vi "Read2 Channels Metodo.vi"(6 "Measurement Type (0: Phase)":i32(ring) items=["Phase", "Delay", "DelayRR", "DelayRF", "DelayFR", "DelayFF"], 8 "error in (no error)":errorcluster, 9 "Channels":T2={"Data Tektronix"={"Channel 1 (1: Channel 1)"=1, "Channel 2 (2: Channel 2)"=2}, "Data Keysight"={"Channels 2"=[], "Timeout (10000 ms)"=10000}} {"Data Keysight"."Channels 2" items=["Channel 1"=0, "Channel 2"=1, "Channel 3"=2, "Channel 4"=3, "Waveform Memory 1"=5, "Waveform Memory 2"=6, "Serial Bus 1"=7, "Serial Bus 2"=8, "Digital Bus Low"=9, "Digital Bus High "=10, "Digital Bus 1"=11, "Digital Bus 2"=12, "External"=29, "Function 1"=32, "Function 2"=33, "Function 3"=34, "Function 4"=35, "Math 1"=36, "Math 2"=37, "Math 3"=38, "Math 4"=39, "FFT"=40, "Analog Bus"=41]; "Data Tektronix"."Channel 2 (2: Channel 2)" items=["Channel 1"=1, "Channel 2"=2, "Channel 3"=3, "Channel 4"=4]; "Data Tektronix"."Channel 1 (1: Channel 1)" items=["Channel 1"=1, "Channel 2"=2, "Channel 3"=3, "Channel 4"=4]}, 11 "Osciloscope in":refnum<class "Osciloscope.lvclass">) -> (0 "error out":errorcluster, 1 "Data Out":T1, 3 "Osciloscope out":refnum<class "Osciloscope.lvclass">)   [LabVIEW 2020, in "Osciloscope.lvclass"]
uses:
  Osciloscope.lvclass
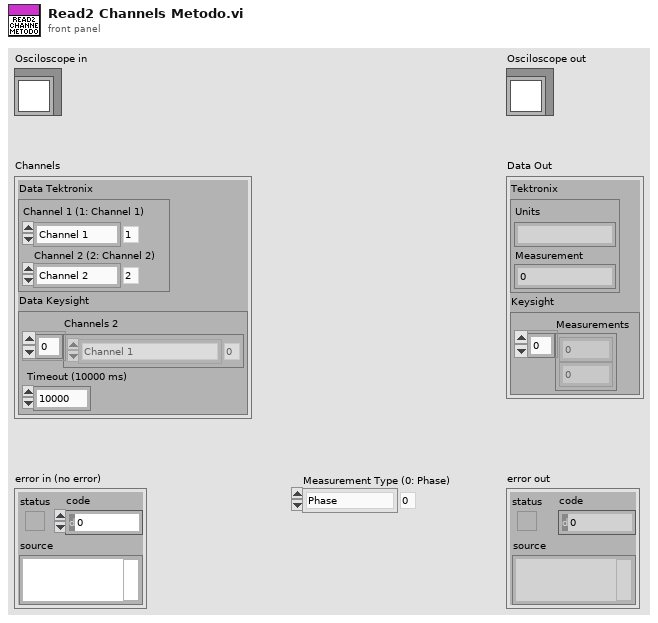
[diagram p1: front panel]
types:
  T1 = cluster{"Tektronix":cluster{"Units":string, "Measurement":dbl}, "Keysight":cluster{"Measurements":dbl[]}}
  T2 = cluster{"Data Tektronix":cluster{"Channel 1 (1: Channel 1)":i32, "Channel 2 (2: Channel 2)":i32}, "Data Keysight":cluster{"Channels 2":i32[], "Timeout (10000 ms)":u32}}
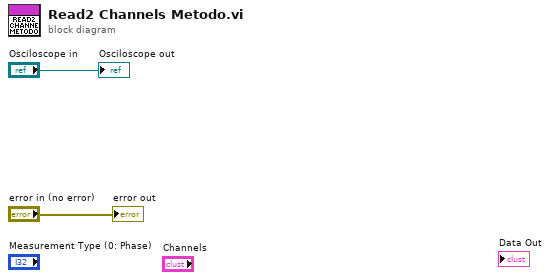
[diagram p0: block diagram]
diagram:
  "Osciloscope out" <- "Osciloscope in"
  "error out" <- "error in (no error)"
